vi "Day 3 - Gear Ratios.vi"() -> ()   [LabVIEW 2020, in "AoC 2023.lvlib"]
uses:
  AoC 2023.lvlib
  <vilib>/Utility/miscctls.llb/LVMapReplaceAction.ctl
panel:
  out "Puzzle Part-2 Answer":string
  out "Puzzle Answer":string
  in  "Puzzle Input":string="467..114..\n...*......\n..35..633.\n......#...\n617*......\n.....+.58.\n..592.....\n......755.\n...$.*....\n.664.598.."
  # "Enter the Puzzle Input and run the VI"
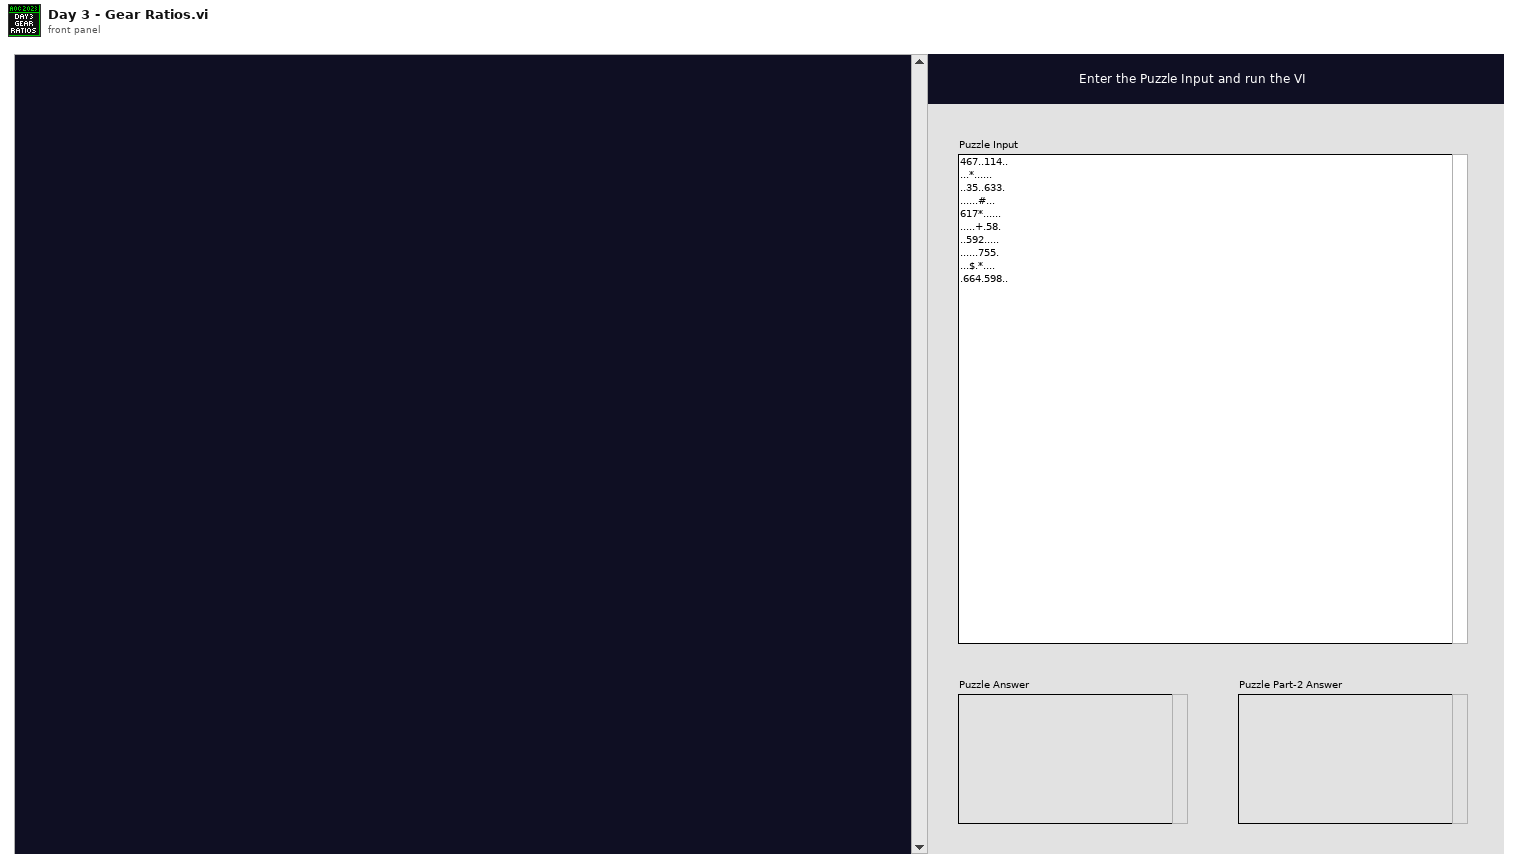
[diagram p1: front panel]
types:
  T1 = typedef "LVMapReplaceAction.ctl" = enum32{"Modify Entry only if found", "Add or Modify Entry", "Delete Entry"}
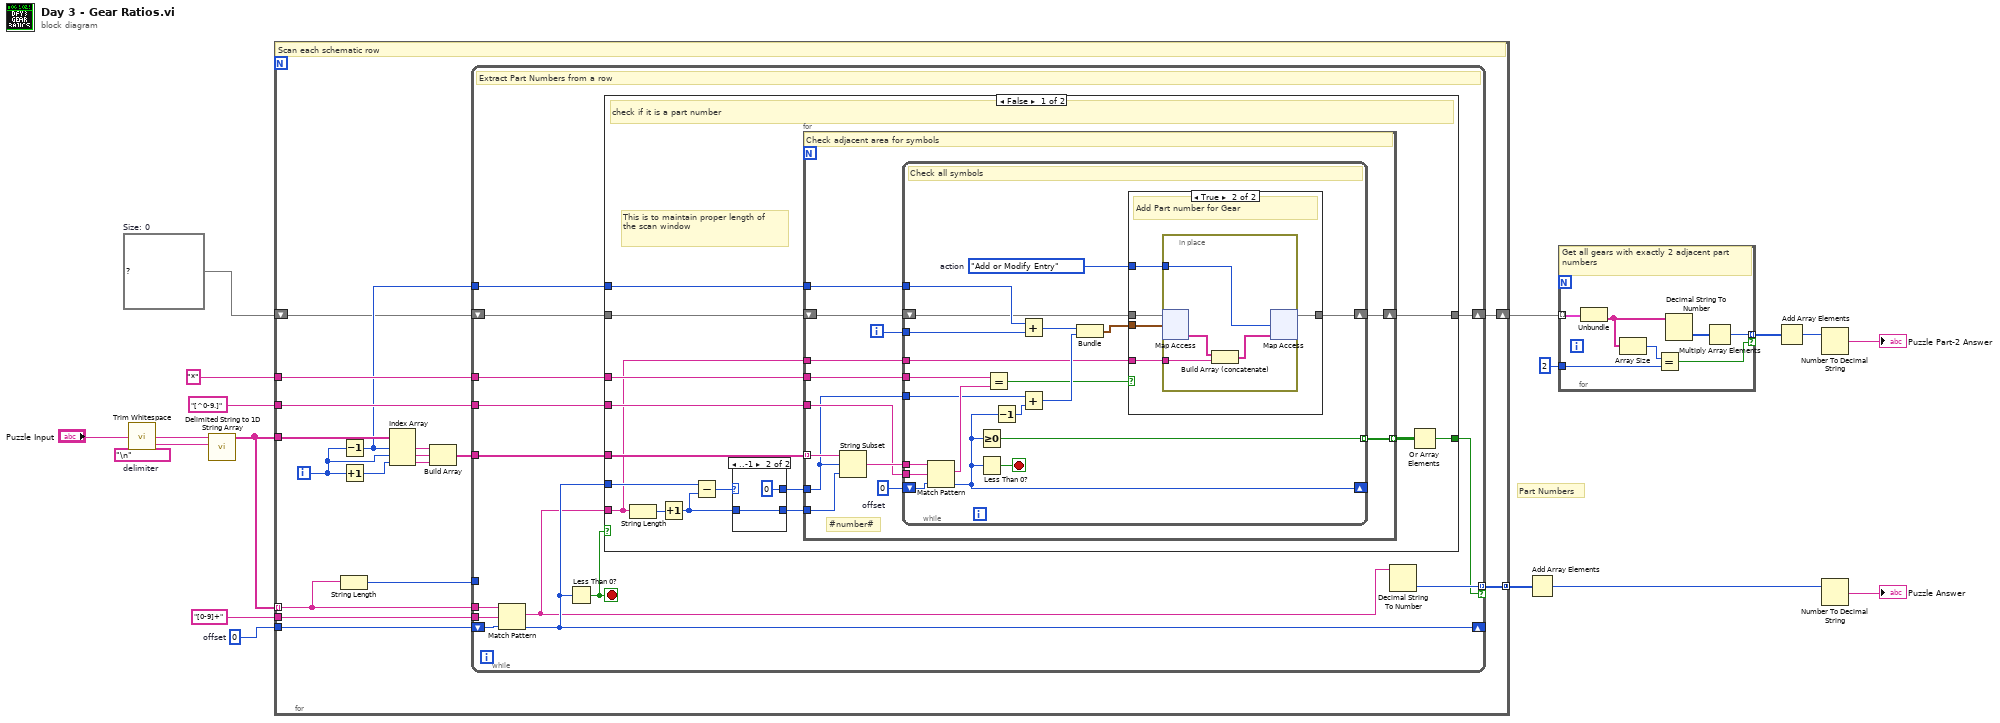
[diagram p0: block diagram]
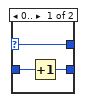
[diagram p2: hidden frame]
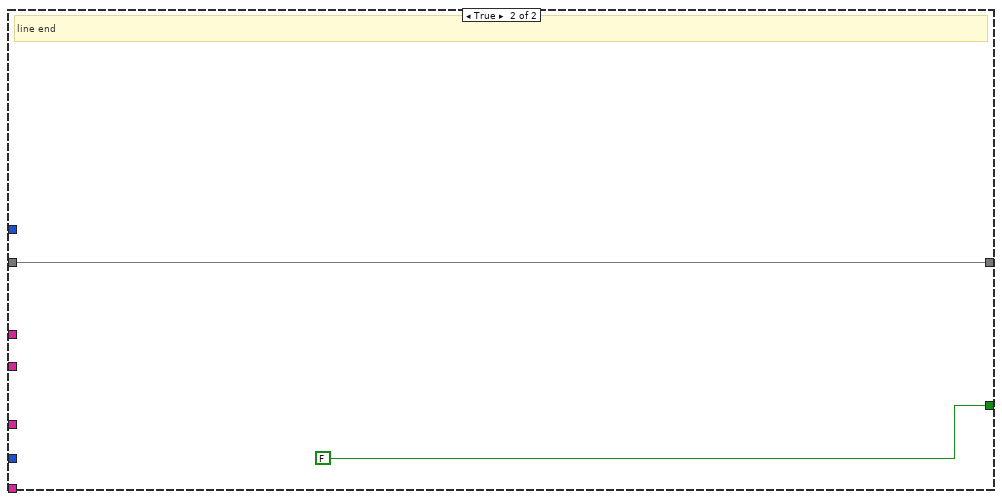
[diagram p4: hidden frame]
diagram:
  w5 = map{cluster{i32, i32}, string[]} {}  # Size: 0
  w10 = 0  # offset
  w14 = "\n"  # delimiter
  # "Part Numbers"
  n1 = call <vilib>:"Trim Whitespace.vi"("string"="Puzzle Input") -> ("trimmed string"=w13:string)  [unwired: 1 in]
  n2 = call <vilib>:"Delimited String to 1D String Array.vi"("delimiter"=w14, "delimited string"=w13) -> ("string array"=w12:string[])  [unwired: 9 in]
  n3 = for {
    tunnel: w12 -> [w23] mode=indexing
    tunnel: w12 -> [w34]
    tunnel: "[0-9]+" -> [w27]
    tunnel: w10 -> [w26]
    tunnel: "[^0-9.]" -> [w25]
    tunnel: [w24] -> w8 mode=concatenating
    tunnel: "*" -> [w21]
    shift-right: [w19] -> w4
    shift-left: w5 -> [w18]
    i -> [w32]
    # "Scan each schematic row"
    n4 = String Length(string=w23) -> (length=w22:i32)
    n5 = Decrement(x=w32) -> (x-1=w20:i32)
    n6 = Increment(x=w32) -> (x+1=w33:i32)
    n7 = Index Array(array=w34, index #1=w20, index #2=w32, index #3=w33) -> (element #1=w31:string, element #2=w30:string, element #3=w29:string)
    n8 = Build Array(w31, w30, w29) -> (w28:string[])
    n9 = while {
      tunnel: w23 -> [w48]
      tunnel: w28 -> [w45]
      shift-right: [w41] -> _
      shift-left: w26 -> [w47]
      tunnel: w27 -> [w46]
      tunnel: w25 -> [w44]
      tunnel: [w43] -> w24 mode=indexing if=w39
      tunnel: w22 -> [_]
      tunnel: w21 -> [w38]
      tunnel: w20 -> [w37]
      shift-right: [w36] -> w19
      shift-left: w18 -> [w35]
      stop <- w42 stop-if-true
      # "Extract Part Numbers from a row"
      n10 = Match Pattern(string=w48, regular expression=w46, offset (0)=w47) -> (match substring=w40:string, offset past match=w41:i32)  [unwired: 2 out]
      n11 = Less Than 0?(x=w41) -> (x < 0?=w42:bool)
      n12 = case shown="False" w42 {
        tunnel: w45 -> [w63 _]
        tunnel: w44 -> [w61 _]
        tunnel: w40 -> [w53 _]
        tunnel: [w57 FALSE] -> w39
        tunnel: w41 -> [w60 _]
        tunnel: w38 -> [w59 _]
        tunnel: w37 -> [w56 _]
        tunnel: [w55 w112] -> w36
        tunnel: w35 -> [w54 w112]
        frame False {
          # "This is to maintain proper length of the scan window"
          # "check if it is a part number"
          n13 = String Length(string=w53) -> (length=w62:i32)
          n14 = Increment(x=w62) -> (x+1=w49:i32)
          n15 = Subtract(x=w60, y=w49) -> (x-y=w52:i32)
          n16 = case shown="..-1" w52 {
            selector: w52 -> [w66 _]
            tunnel: [w66 0] -> w51
            tunnel: [w65 w67] -> w50
            tunnel: w49 -> [w64 w67]
            frame 0.. {
              n17 = Increment(x=w64) -> (x+1=w65:i32)
            }
            frame ..-1 {
            }
          }
          n18 = for {
            tunnel: w63 -> [w81] mode=indexing
            tunnel: w51 -> [w74]
            tunnel: w50 -> [w80]
            tunnel: w61 -> [w78]
            tunnel: [w77] -> w58 mode=indexing
            tunnel: w59 -> [w76]
            tunnel: w56 -> [w73]
            shift-right: [w72] -> w55
            shift-left: w54 -> [w71]
            tunnel: w53 -> [w70]
            i -> [w69]
            w75 = 0  # offset
            # "#number#"
            # "Check adjacent area for symbols"
            n19 = String Subset(string=w81, offset (0)=w74, length (rest)=w80) -> (substring=w79:string)
            n20 = while {
              tunnel: w79 -> [w101]
              tunnel: w78 -> [w100]
              tunnel: [w99] -> w77 mode=indexing
              tunnel: w76 -> [w98]
              shift-right: [w94] -> _
              shift-left: w75 -> [w96]
              tunnel: w74 -> [w92]
              tunnel: w73 -> [w91]
              shift-right: [w87] -> w72
              shift-left: w71 -> [w86]
              tunnel: w70 -> [w85]
              tunnel: w69 -> [w82]
              stop <- w95 stop-if-true
              w84 = LVMapReplaceAction."Add or Modify Entry"  # action
              # "Check all symbols"
              n21 = Match Pattern(string=w101, regular expression=w100, offset (0)=w96) -> (match substring=w97:string, offset past match=w94:i32)  [unwired: 2 out]
              n22 = Greater Or Equal To 0?(x=w94) -> (x >= 0?=w99:bool)
              n23 = Less Than 0?(x=w94) -> (x < 0?=w95:bool)
              n24 = Equal?(x=w98, y=w97) -> (x = y?=w83:bool)
              n25 = Decrement(x=w94) -> (x-1=w93:i32)
              n26 = Add(x=w91, y=w82) -> (x+y=w90:i32)
              n27 = Add(x=w92, y=w93) -> (x+y=w89:i32)
              n28 = Bundle(w90, w89) -> (w88:cluster{i32, i32})  [unwired: 1 in]
              n29 = case shown="True" w83 {
                tunnel: w88 -> [_ w107]
                tunnel: [w102 w106] -> w87
                tunnel: w86 -> [w102 w105]
                tunnel: w85 -> [_ w104]
                tunnel: w84 -> [_ w103]
                frame False {
                }
                frame True {
                  # "Add Part number for Gear"
                  n30 = in-place {
                    in-place-border: w104 -> [w111]
                    in-place-border: w103 -> [w108]
                    n31 = in-place-map #1(w105, w107) -> (w109:string[])  [unwired: 1 in, 1 out]
                    n32 = Build Array (concatenate)(w109, w111) -> (w110:string[])
                    n33 = in-place-map #1(w110, w108) -> (w106:map{cluster{i32, i32}, string[]})  [unwired: 2 out]
                  }
                }
              }
            }
          }
          n34 = Or Array Elements(Boolean array=w58) -> (logical OR=w57:bool)
        }
        frame True {
          # "line end"
        }
      }
      n35 = Decimal String To Number(string=w40) -> (number=w43:i32)  [unwired: 2 in, 1 out]
    }
  }
  n36 = Add Array Elements(numeric array=w8) -> (sum=w7:i32)
  n37 = for {
    tunnel: w4 -> [w120] mode=indexing
    tunnel: [w117] -> w3 mode=indexing if=w115
    tunnel: 2 -> [w114]
    # "Get all gears with exactly 2 adjacent part numbers"
    n38 = Unbundle(w120) -> (w116:string[])  [unwired: 1 out]
    n39 = Array Size(array=w116) -> (size(s)=w119:i32)
    n40 = Equal?(x=w119, y=w114) -> (x = y?=w115:bool)
    n41 = Decimal String To Number(string=w116) -> (number=w118:i32[])  [unwired: 2 in, 1 out]
    n42 = Multiply Array Elements(1:w118) -> (0:w117:i32)
  }
  n43 = Add Array Elements(numeric array=w3) -> (sum=w2:i32)
  n44 = Number To Decimal String(number=w2) -> (decimal integer string=→"Puzzle Part-2 Answer":string)  [unwired: 1 in]
  n45 = Number To Decimal String(number=w7) -> (decimal integer string=→"Puzzle Answer":string)  [unwired: 1 in]
